vi "Write aVar Params.vi"(8 "error in (no error)":errorcluster, 10 "aVar Params":T1={"tmeas"=0.001, "tint"=[0.001, 0.01, 0.1, 1.0, 3.0], "ttot"=15.0, "Varaince On"=FALSE}, 11 "CRDS Cell in":refnum<class "CRDS Cell.lvclass">) -> (0 "error out":errorcluster, 3 "CRDS Cell out":refnum<class "CRDS Cell.lvclass">)   [LabVIEW 2012, in "CRDS Cell.lvclass"]
uses:
  CRDS Cell.lvclass
  CRDS Cell.lvclass/CRDS Cell.ctl
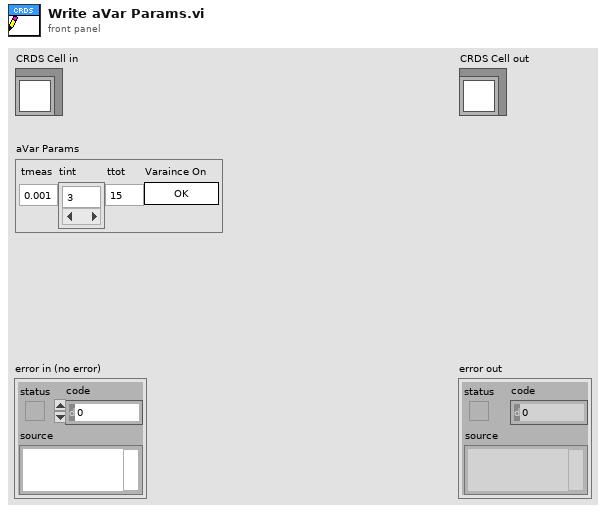
[diagram p1: front panel]
types:
  T1 = cluster{"tmeas":dbl, "tint":sgl[], "ttot":dbl, "Varaince On":bool}
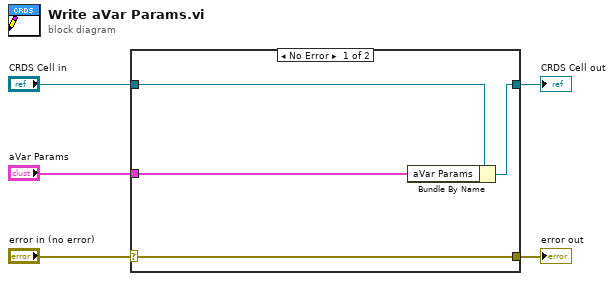
[diagram p0: block diagram]
diagram:
  n1 = case shown="No Error" "error in (no error)" {
    selector: "error in (no error)" -> [w9 w10]
    tunnel: [w9 w10] -> w4
    tunnel: [w7 w11] -> w2
    tunnel: "CRDS Cell in" -> [w8 w11]
    tunnel: "aVar Params" -> [w6 _]
    frame No Error {
      n2 = Bundle By Name(cluster=w8, "aVar Params"=w6) -> (w7:refnum<class "CRDS Cell.lvclass">)
    }
    frame Error {
    }
  }
  "error out" <- w4
  "CRDS Cell out" <- w2
